vi "Axis.vi"(1 "Color":u32(colorbox), 2 "Alpha":dbl=1.0, 3 "Half plane?":bool=TRUE, 5 "Name":string="XYZ axis", 7 "Length":sgl=2.0, 9 "Radius":sgl=0.01, 11 "error in (no error)":errorcluster, 12 "Axis label?":bool, 13 "Character Size":sgl=0.5) -> (4 "3D Object out":refnum<class "3D Object.lvclass">, 15 "error out":errorcluster)   [LabVIEW 2015, in "3D Object.lvclass"]
uses:
  3D Object.lvclass
  3D Object.lvclass/3D Object.ctl
  <vilib>/picture/3D Picture Control/NI_3D Picture Control.lvlib
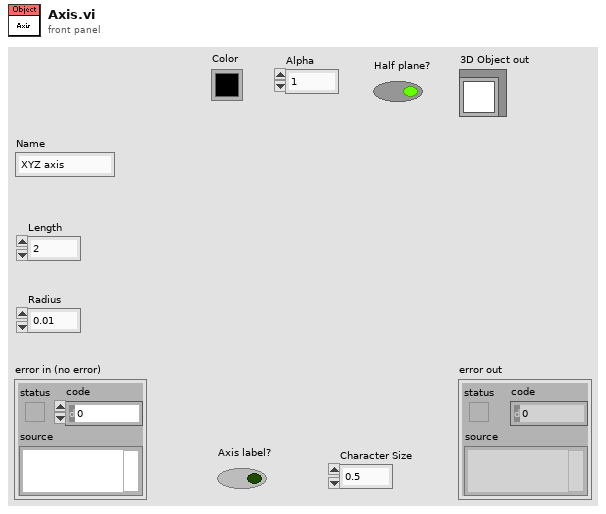
[diagram p1: front panel]
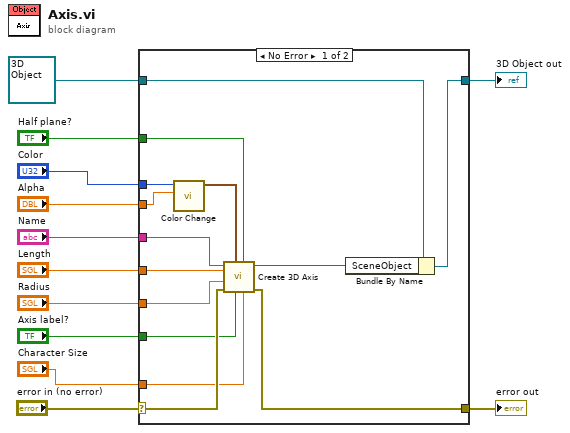
[diagram p0: block diagram]
diagram:
  n1 = case shown="No Error" "error in (no error)" {
    selector: "error in (no error)" -> [w21 w28]
    tunnel: [w20 w28] -> w11
    tunnel: [w13 w27] -> w9
    tunnel: refnum<class "3D Object.lvclass"> refnum ("3D Object in") -> [w25 w27]
    tunnel: "Name" -> [w24 _]
    tunnel: "Length" -> [w23 _]
    tunnel: "Radius" -> [w22 _]
    tunnel: "Color" -> [w18 _]
    tunnel: "Alpha" -> [w17 _]
    tunnel: "Axis label?" -> [w16 _]
    tunnel: "Half plane?" -> [w15 _]
    tunnel: "Character Size" -> [w14 _]
    frame No Error {
      n2 = call <vilib>:"Color Change.vi"("Alpha"=w17, "Color"=w18) -> ("RGBA"=w19:cluster{"R":sgl, "G":sgl, "B":sgl, "A":sgl})  [unwired: 9 out]
      n3 = call <vilib>:"Create 3D Axis.vi"("Character Size"=w14, "Half plane?"=w15, "Axis label?"=w16, "Color"=w19, "error in (no error)"=w21, "Radius"=w22, "Length"=w23, "Name"=w24) -> ("error out"=w20:errorcluster, "New Object Refnum"=w26:refnum<vi>)  [unwired: 2 in]
      n4 = Bundle By Name(cluster=w25, "SceneObject"=w26) -> (w13:refnum<class "3D Object.lvclass">)
    }
    frame Error {
    }
  }
  "error out" <- w11
  "3D Object out" <- w9
